vi "P4CMD Check Out.vi"(7 "advanced options":variant, 8 "error in (no error)":errorcluster, 9 "comment":string, 10 "files":path[](array[path]), 11 "source control reference in":T1) -> (0 "error out":errorcluster, 1 "dialog box cancelled?":bool, 2 "status message":string, 3 "source control reference out":T1)   [LabVIEW 2020, in "NI_SCC_P4CMD.lvlib"]
uses:
  <vilib>/SourceControl/Providers/P4CMD/NI_SCC_P4CMD.lvlib
  <vilib>/SourceControl/sccapi/SCCAPI Refnum.ctl
  <vilib>/SourceControl/Providers/P4CMD/P4CMD Mgr Functions.ctl
  <vilib>/SourceControl/sccapi/SCCAPI Get Retrieval Method.ctl
  <vilib>/SourceControl/Providers/P4CMD/P4CMD Operations.ctl
  <vilib>/SourceControl/support/SCCSup Message Strings GLBL.vi
  <vilib>/SourceControl/sccapi/NI_SCC.lvlib
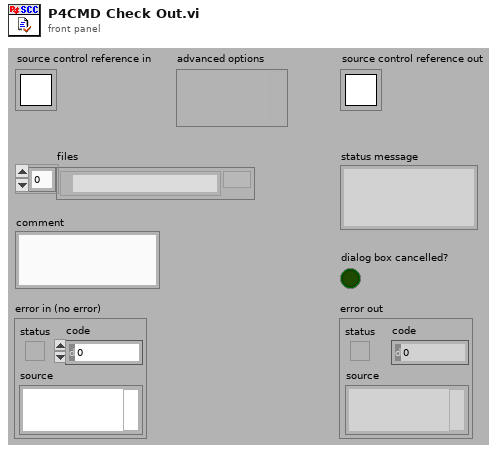
[diagram p1: front panel]
types:
  T1 = typedef "NI_SCC.lvlib/SCCAPI Refnum.ctl" = refnum<k1>
  T2 = typedef "NI_SCC_P4CMD.lvlib/P4CMD Mgr Functions.ctl" = enum16{"Init", "Open", "Set Config Opts", "Initialized?", "IsRefValid?", "Get Config Opts", "Get Global Commands", "Close", "Uninit"}
  T3 = enum16{"Left Button", "Center Button", "Right Button", "Window Close"}
  T4 = cluster{"Left Button Key Shortcut":cluster{"Control":bool, "Shift":bool, "Key":string}, "Center Button Key Shortcut":cluster{"Control":bool, "Shift":bool, "Key":string}, "Right Button Key Shortcut":cluster{"Control":bool, "Shift":bool, "Key":string}}
  T5 = typedef "NI_SCC_P4CMD.lvlib/P4CMD Operations.ctl" = enum16{"get all clients", "get all users", "describe changelist", "sync from depot", "open for edit", "submit to depot", "revert", "add to depot", "remove from depot", "print files revisions", "compare client file", "print depot file contents", "list opened files", "get file info", "lock files", "edit changelist spec", "info", "set variables"}
  T6 = typedef "NI_SCC_P4CMD.lvlib/P4CMD Advanced Options.ctl" = cluster{"lock files?":bool, "suppress dialogs?":bool}
  T7 = typedef "NI_SCC.lvlib/SCCAPI SCC File Status.ctl" = cluster{"in source control?":bool, "checked out by user?":bool, "checked out by other?":bool, "out of date?":bool, "deleted?":bool}
  T8 = typedef "NI_SCC.lvlib/SCCAPI Get Retrieval Method.ctl" = u16
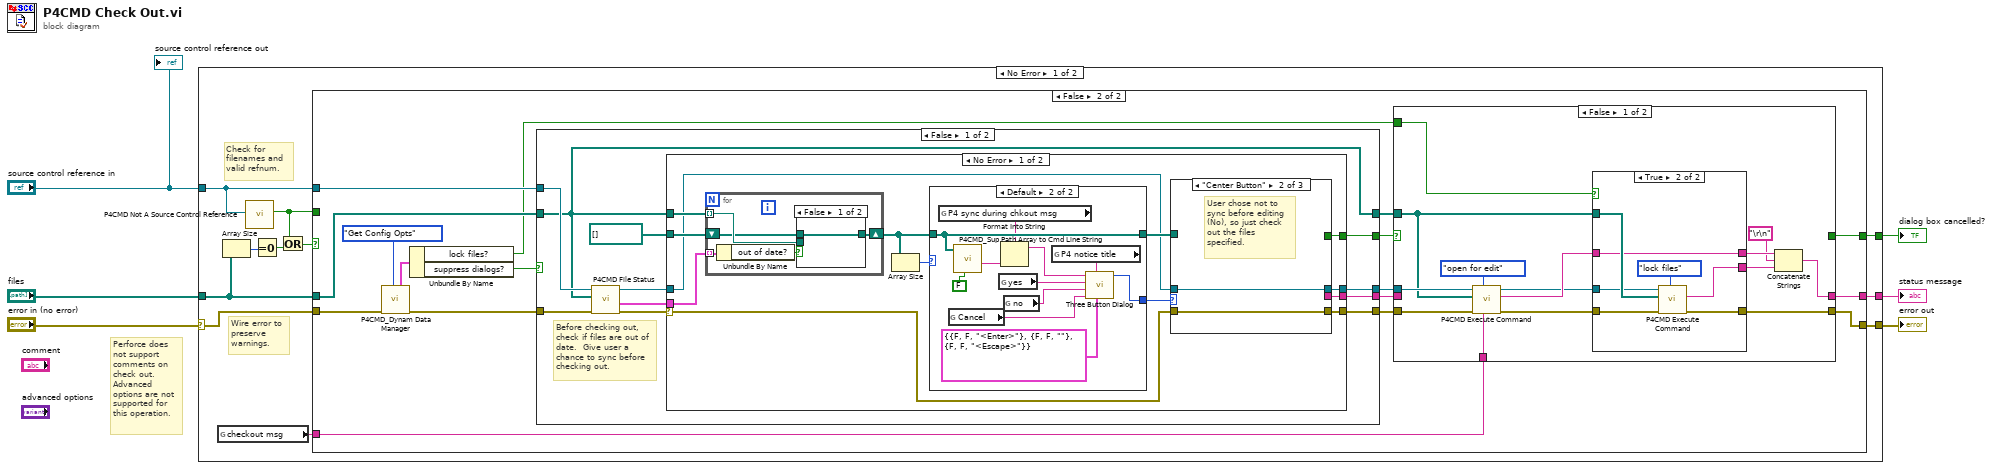
[diagram p0: block diagram]
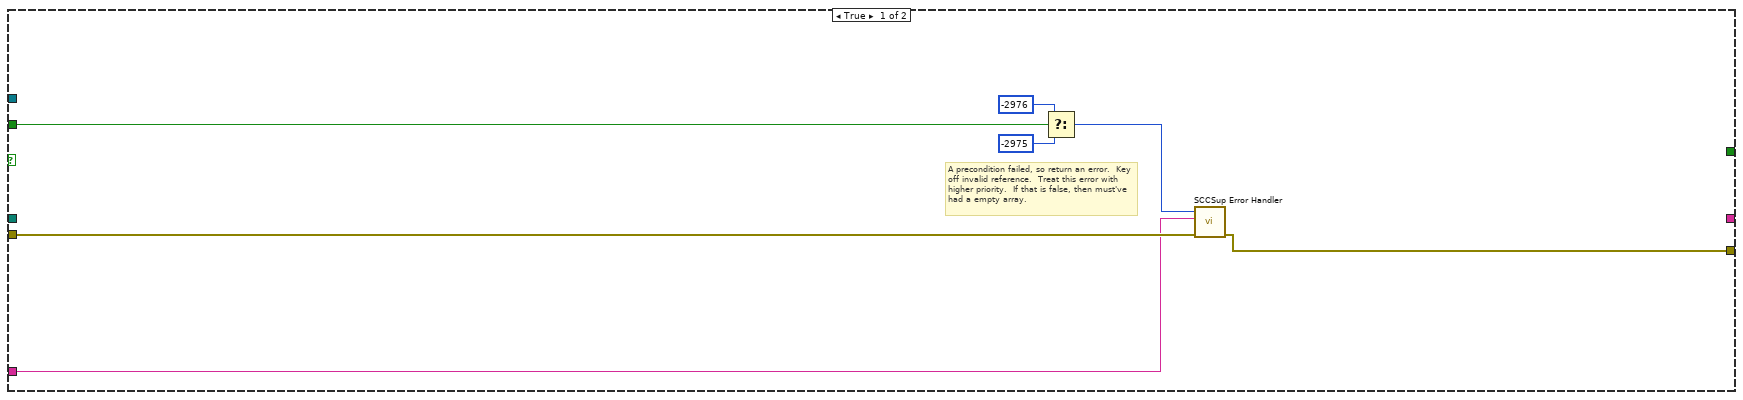
[diagram p2: hidden frame]
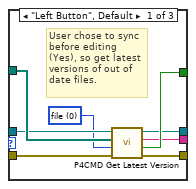
[diagram p3: hidden frame]
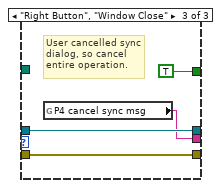
[diagram p4: hidden frame]
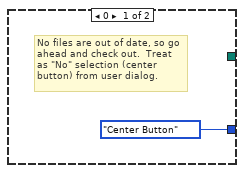
[diagram p5: hidden frame]
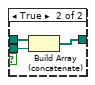
[diagram p6: hidden frame]
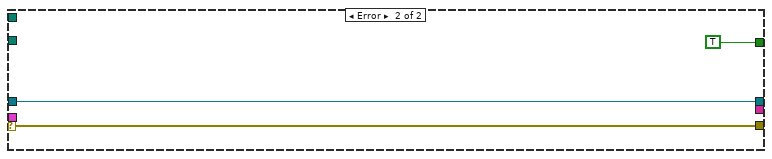
[diagram p7: hidden frame]
diagram:
  # "Perforce does not support comments on check out.  Advanced options are not supported for this operation."
  n1 = case shown="No Error" "error in (no error)" {
    selector: "error in (no error)" -> [w9 w133]
    tunnel: [w7 w133] -> w5
    tunnel: "source control reference in" -> [w14 _]
    tunnel: [w17 _] -> w3
    tunnel: "files" -> [w13 _]
    tunnel: [w10 _] -> w1
    frame No Error {
      # "Wire error to preserve warnings."
      # "Check for filenames and valid refnum."
      n2 = global read "SCCSup Message Strings GLBL.vi" "checkout msg"() -> (w8:string)
      n3 = Array Size(array=w13) -> (size(s)=w16:i32)
      n4 = call <vilib>:"P4CMD Not A Source Control Reference.vi"("source control reference in"=w14) -> ("not a source control reference?"=w11:bool)  [unwired: 9 in, 1 out]
      n5 = Equal To 0?(x=w16) -> (x = 0?=w15:bool)
      n6 = Or(x=w11, y=w15) -> (x .or. y?=w12:bool)
      n7 = case shown="False" w12 {
        tunnel: w14 -> [_ w29]
        tunnel: [_ w35] -> w17
        tunnel: w13 -> [_ w38]
        tunnel: w11 -> [w22 _]
        tunnel: [_ w36] -> w10
        tunnel: w9 -> [w19 w28]
        tunnel: w8 -> [w18 w33]
        tunnel: [w21 w34] -> w7
        frame True {
          # "A precondition failed, so return an error.  Key off invalid reference.  Treat this error with higher priority.  If that is false, then must've had a empty array."
          n8 = Select(t=-2976 ("result"), s=w22, f=-2975 ("result")) -> (s? t:f=w20:i32)
          n9 = call <vilib>:"SCCSup Error Handler.vi"("error in (no error)"=w19, "operation message"=w18, "scc error code"=w20) -> ("error out"=w21:errorcluster)  [unwired: 8 in]
        }
        frame False {
          n10 = call <vilib>:"P4CMD_Dynam Data Manager.vi"("function"=P4CMD_Mgr_Functions."Get Config Opts", "error in (no error)"=w28) -> ("error out"=w27:errorcluster, "adv cfg options out"=w31:T6)  [unwired: 4 in, 4 out]
          n11 = Unbundle By Name(w31) -> ("lock files?"=w25:bool, "suppress dialogs?"=w30:bool)
          n12 = case shown="False" w30 {
            tunnel: w27 -> [w52 w106]
            tunnel: [w48 w106] -> w41
            tunnel: [w47 _] -> w40
            tunnel: [w46 _] -> w39
            tunnel: w38 -> [w42 w104]
            tunnel: [w45 w105] -> w37
            tunnel: w29 -> [w43 w105]
            tunnel: [w42 w104] -> w26
            frame False {
              # "Before checking out, check if files are out of date.  Give user a chance to sync before checking out."
              n13 = call <vilib>:"P4CMD File Status.vi"("error in (no error)"=w52, "files"=w42, "source control reference in"=w43) -> ("error out"=w49:errorcluster, "file status"=w51:T7[], "source control reference out"=w44:T1)  [unwired: 4 in, 2 out]
              n14 = case shown="No Error" w49 {
                selector: w49 -> [w53 w103]
                tunnel: w51 -> [w65 _]
                tunnel: w42 -> [w64 _]
                tunnel: path[] [] -> [w63 _]
                tunnel: [w58 w103] -> w48
                tunnel: [w55 w101] -> w45
                tunnel: [w57 _] -> w46
                tunnel: [w56 TRUE ("dialog box cancelled?")] -> w47
                tunnel: w44 -> [w54 w101]
                frame No Error {
                  n15 = for {
                    tunnel: w65 -> [w96] mode=indexing
                    tunnel: w64 -> [w94] mode=indexing
                    shift-right: [w93] -> w61
                    shift-left: w63 -> [w92]
                    n16 = Unbundle By Name(w96) -> ("out of date?"=w95:bool)
                    n17 = case shown="False" w95 {
                      tunnel: w94 -> [_ w100]
                      tunnel: [w97 w99] -> w93
                      tunnel: w92 -> [w97 w98]
                      frame False {
                      }
                      frame True {
                        n18 = Build Array (concatenate)(w98, w100) -> (w99:path[])
                      }
                    }
                  }
                  n19 = Array Size(array=w61) -> (size(s)=w62:i32)
                  n20 = case shown="Default" w62 {
                    tunnel: w61 -> [_ w90]
                    tunnel: [T3."Center Button" ("Which Button?") w88] -> w60
                    tunnel: [_ w90] -> w59
                    frame 0 {
                      # "No files are out of date, so go ahead and check out.  Treat as \"No\" selection (center button) from user dialog."
                    }
                    frame Default {
                      n21 = global read "SCCSup Message Strings GLBL.vi" "P4 sync during chkout msg"() -> (w89:string)
                      n22 = global read "SCCSup Message Strings GLBL.vi" "Cancel"() -> (w83:string)
                      n23 = call <vilib>:"P4CMD_Sup Path Array to Cmd Line String.vi"("expand wildcards? (T)"=FALSE, "files"=w90) -> ("string output"=w91:string)  [unwired: 8 in, 1 out]
                      n24 = global read "SCCSup Message Strings GLBL.vi" "yes"() -> (w85:string)
                      n25 = Format Into String(format string=w89, w91) -> (resulting string=w86:string)  [unwired: 2 in, 1 out]
                      n26 = global read "SCCSup Message Strings GLBL.vi" "no"() -> (w84:string)
                      n27 = global read "SCCSup Message Strings GLBL.vi" "P4 notice title"() -> (w87:string)
                      n28 = call <vilib>:"Three Button Dialog.vi"("Keyboard Shortcuts (Left is <Enter>)"=T4 {"Left Button Key Shortcut"={"Control"=FALSE, "Shift"=FALSE, "Key"="<Enter>"}, "Center Button Key Shortcut"={"Control"=FALSE, "Shift"=FALSE, "Key"=""}, "Right Button Key Shortcut"={"Control"=FALSE, "Shift"=FALSE, "Key"="<Escape>"}}, "Window Title (\"\")"=w87, "Right Button Text (\"Cancel\")"=w83, "Center Button Text (\"No\")"=w84, "Left Button Text (\"Yes\")"=w85, "message"=w86) -> ("Which Button?"=w88:T3)  [unwired: 5 in]
                    }
                  }
                  n29 = case shown="\"Center Button\"" w60 {
                    tunnel: w53 -> [w71 w74 w77]
                    tunnel: w59 -> [w73 _ _]
                    tunnel: w54 -> [w72 w75 w78]
                    tunnel: [w70 w74 w77] -> w58
                    tunnel: [w69 _ TRUE ("dialog box cancelled?")] -> w56
                    tunnel: [w68 w75 w78] -> w55
                    tunnel: [w67 _ w76] -> w57
                    frame "Left Button", Default {
                      w66 = T8 0 items=["file", "directory", "directory (recursive)"] ("retrieval method (file)")
                      # "User chose to sync before editing (Yes), so get latest versions of out of date files."
                      n30 = call <vilib>:"P4CMD Get Latest Version.vi"("error in (no error)"=w71, "retrieval method (file)"=w66, "files"=w73, "source control reference in"=w72) -> ("error out"=w70:errorcluster, "dialog box cancelled?"=w69:bool, "status message"=w67:string, "source control reference out"=w68:T1)  [unwired: 4 in]
                    }
                    frame "Center Button" {
                      # "User chose not to sync before editing (No), so just check out the files specified."
                    }
                    frame "Right Button", "Window Close" {
                      # "User cancelled sync dialog, so cancel entire operation."
                      n31 = global read "SCCSup Message Strings GLBL.vi" "P4 cancel sync msg"() -> (w76:string)
                    }
                  }
                }
                frame Error {
                }
              }
            }
            frame True {
              # "Don't show sync helper dialog.  Just check out the specified files."
            }
          }
          n32 = case shown="False" w40 {
            selector: w40 -> [_ w132]
            tunnel: w41 -> [w118 w130]
            tunnel: w39 -> [_ w131]
            tunnel: w26 -> [w113 _]
            tunnel: w37 -> [w114 _]
            tunnel: [_ w132] -> w36
            tunnel: [w116 w131] -> w35
            tunnel: [w120 w130] -> w34
            tunnel: w33 -> [w109 _]
            tunnel: w25 -> [w107 _]
            frame False {
              n33 = call <vilib>:"P4CMD Execute Command.vi"("operation message"=w109, "p4 operation"=P4CMD_Operations."open for edit", "error in (no error)"=w118, "files"=w113, "source control reference in"=w114) -> ("error out"=w117:errorcluster, "command information"=w115:string, "source control reference out"=w108:T1)  [unwired: 4 in]
              n34 = case shown="True" w107 {
                tunnel: w117 -> [w122 w128]
                tunnel: [w122 w127] -> w120
                tunnel: w115 -> [w121 w125]
                tunnel: w113 -> [_ w126]
                tunnel: [w121 w125] -> w112
                tunnel: [_ w124] -> w111
                tunnel: w108 -> [_ w123]
                frame False {
                }
                frame True {
                  n35 = call <vilib>:"P4CMD Execute Command.vi"("p4 operation"=P4CMD_Operations."lock files", "error in (no error)"=w128, "files"=w126, "source control reference in"=w123) -> ("error out"=w127:errorcluster, "command information"=w124:string)  [unwired: 5 in, 1 out]
                }
              }
              n36 = Concatenate Strings(w112, "\r\n", w111) -> (w116:string)
            }
            frame True {
            }
          }
        }
      }
    }
    frame Error {
    }
  }
  "error out" <- w5
  "status message" <- w3
  "dialog box cancelled?" <- w1
  "source control reference out" <- "source control reference in"
